vi "Check Read_Write.vi"(8 "error in (no error)":errorcluster, 11 "Simulation in":refnum<class "Simulation.lvclass">) -> (0 "error out":errorcluster, 3 "Simulation out":refnum<class "Simulation.lvclass">)   [LabVIEW 2020, in "Generic I2C.lvlib" / "Simulation.lvclass"]
uses:
  Simulation.lvclass
  C:/Users/kaiser.asan/OneDrive - SolitonTechnologies/LabVIEW/29.SDLC - I2C Driver/I2C Module/I2C Controller Module/Class/Devices/Parent/Devices.lvclass
  Transmission Mode/Parent/TX Speed.lvclass
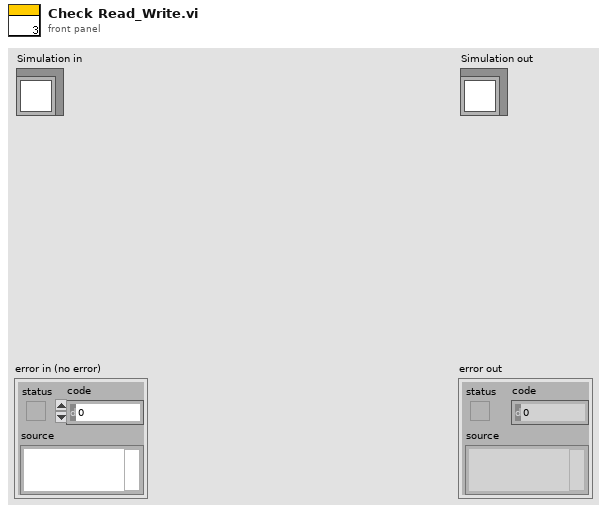
[diagram p1: front panel]
types:
  T1 = typedef "I2C Controller Lib.lvlib/Transmission Data.ctl" = u8[]
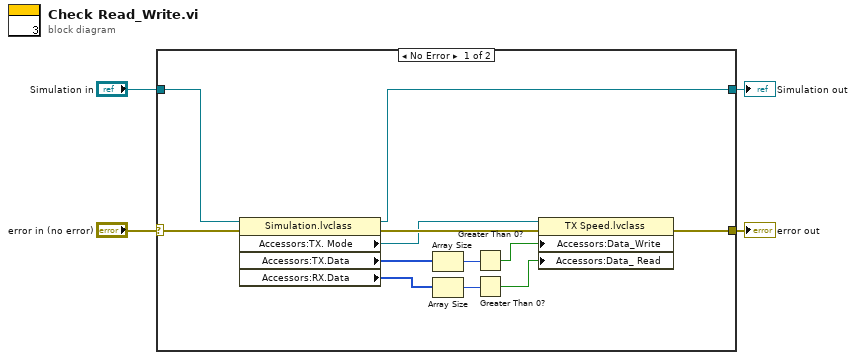
[diagram p0: block diagram]
diagram:
  n1 = case shown="No Error" "error in (no error)" {
    selector: "error in (no error)" -> [w16 w17]
    tunnel: [w11 w18] -> w4
    tunnel: "Simulation in" -> [w14 w18]
    tunnel: [w13 w17] -> w2
    frame No Error {
      n2 = property class="Simulation.lvclass"(reference=w14, error in=w16) -> (reference out=w11:refnum<class "Simulation.lvclass">, error out=w15:errorcluster, "Accessors:TX. Mode"=w12:refnum<data-value>, "Accessors:TX.Data"=w9:T1, "Accessors:RX.Data"=w6:u8[])
      n3 = Array Size(array=w9) -> (size(s)=w10:i32)
      n4 = Array Size(array=w6) -> (size(s)=w7:i32)
      n5 = Greater Than 0?(x=w10) -> (x > 0?=w8:bool)
      n6 = Greater Than 0?(x=w7) -> (x > 0?=w5:bool)
      n7 = property class="TX Speed.lvclass"(reference=w12, error in=w15, "Accessors:Data_Write"=w8, "Accessors:Data_ Read"=w5) -> (error out=w13:errorcluster)  [unwired: 1 out]
    }
    frame Error {
    }
  }
  "error out" <- w2
  "Simulation out" <- w4
